vi "Read Settings.vi"(0 "Sequence File Path":path, 5 "Charact type":string="Scalar", 7 "Use Operator Mode":bool=TRUE, 11 "error in":errorcluster) -> (4 "Config File Path":path, 6 "Silent Option Enabled?":bool, 8 "Check Path Expiration?":bool=TRUE, 10 "Use command-line?":bool=TRUE, 13 "Charact By Standard?":bool, 14 "Setting Section Exists?":bool, 15 "error out":errorcluster)   [LabVIEW 2023, in "RFFixtureCharact.Public.lvlib"]
uses:
  RFFixtureCharact.Public.lvlib
  Common/Data Cache/Settings Dictionary/Setting Keys.vi
  Common/RFCalAndFixtureCharact.Common.lvlib
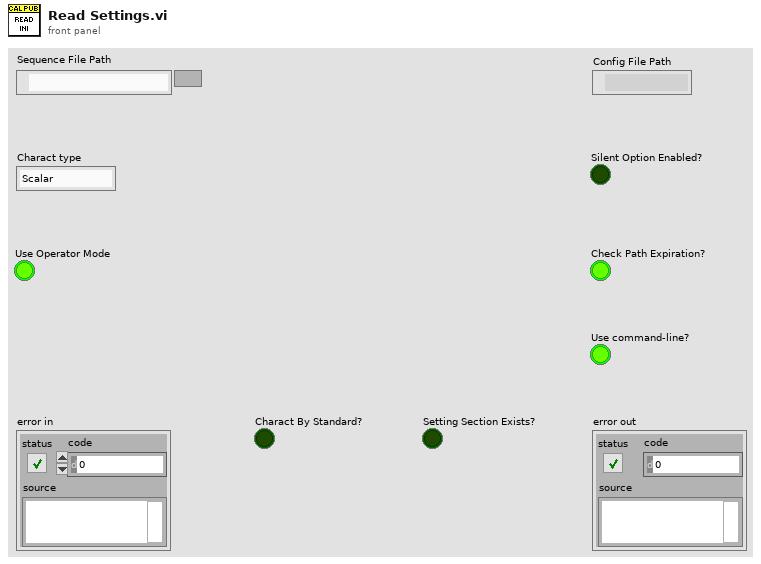
[diagram p1: front panel]
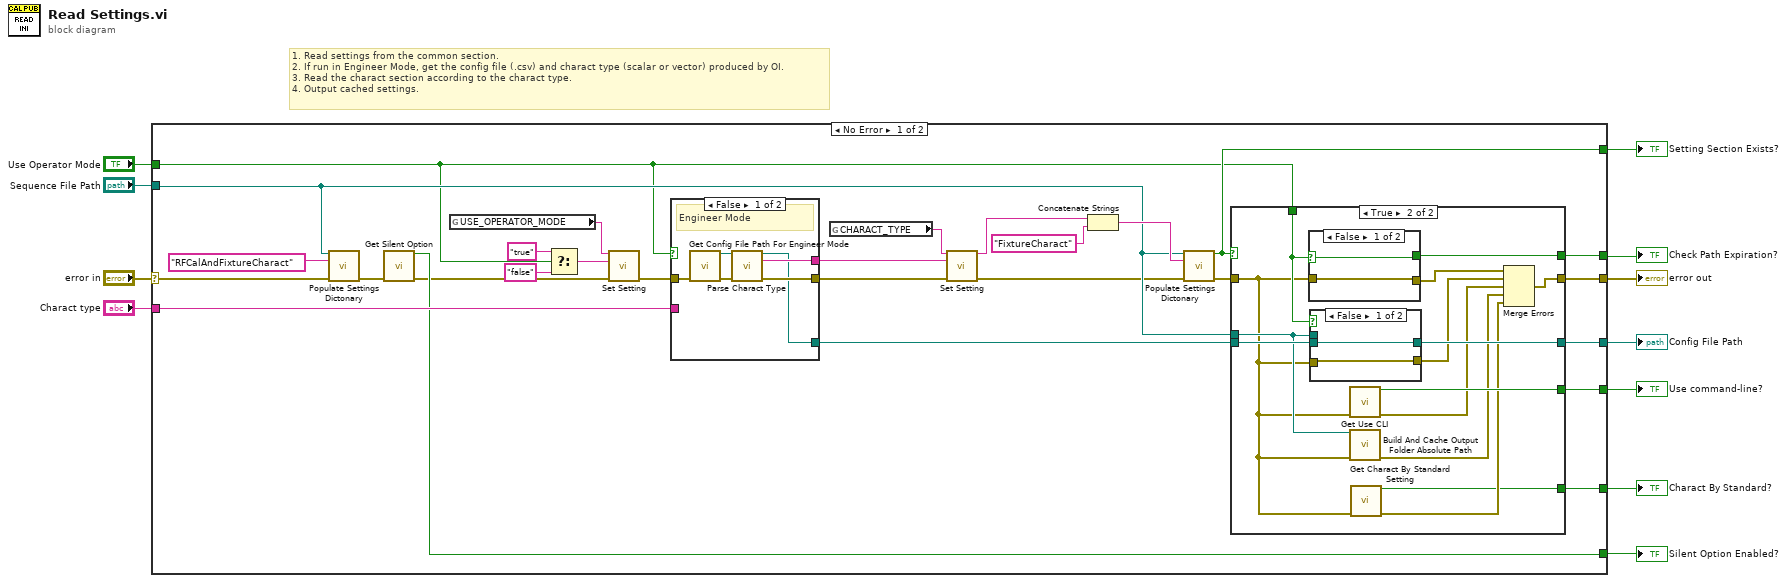
[diagram p0: block diagram]
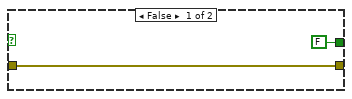
[diagram p2: hidden frame]
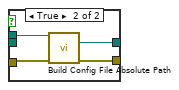
[diagram p3: hidden frame]
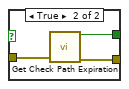
[diagram p4: hidden frame]
diagram:
  # "1. Read settings from the common section.\n2. If run in Engineer Mode, get the config file (.csv) and charact type (scalar or vector) produced by OI.\n3. Read the charact section according to the charact type.\n4. Output cached settings."
  n1 = case shown="No Error" "error in" {
    selector: "error in" -> [w35 w75]
    tunnel: "Charact type" -> [w34 _]
    tunnel: [w19 _] -> w9
    tunnel: [w32 _] -> w8
    tunnel: [w31 _] -> w7
    tunnel: "Sequence File Path" -> [w26 _]
    tunnel: [w30 w75] -> w5
    tunnel: [w33 _] -> w4
    tunnel: [w21 _] -> w3
    tunnel: [w20 _] -> w2
    tunnel: "Use Operator Mode" -> [w15 _]
    frame No Error {
      n2 = call "Populate Settings Dictonary.vi"("sequence file path"=w26, "Section Name"="RFCalAndFixtureCharact", "error in (no error)"=w35) -> ("error out"=w38:errorcluster)  [unwired: 11 in, 1 out]
      n3 = call "Get Silent Option.vi"("error in (no error)"=w38) -> ("Silent Option Enabled?"=w19:bool, "error out"=w18:errorcluster)  [unwired: 13 in]
      n4 = global read "Setting Keys.vi" "USE_OPERATOR_MODE"() -> (w16:string)
      n5 = Select(t="true" ("Section Name"), s=w15, f="false") -> (s? t:f=w12:string)
      n6 = call "Set Setting.vi"("Setting name"=w16, "Setting value"=w12, "error in (no error)"=w18) -> ("error out"=w17:errorcluster)  [unwired: 10 in, 2 out]
      n7 = case shown="False" w15 {
        tunnel: w17 -> [w70 w73]
        tunnel: [w72 w73] -> w36
        tunnel: [w71 w74] -> w24
        tunnel: w34 -> [_ w74]
        tunnel: [w68 _] -> w29
        frame False {
          # "Engineer Mode"
          n8 = call "Get Config File Path For Engineer Mode.vi"("error in (no error)"=w70) -> ("Config File Path"=w67:path, "error out"=w69:errorcluster)  [unwired: 13 in]
          n9 = call "Parse Charact Type.vi"("Config File in"=w67, "error in (no error)"=w69) -> ("Config File out"=w68:path, "Charact type (scalar or vector)"=w71:string, "error out"=w72:errorcluster)  [unwired: 11 in]
        }
        frame True {
          # "Operator Mode"
        }
      }
      n10 = global read "Setting Keys.vi" "CHARACT_TYPE"() -> (w22:string)
      n11 = call "Set Setting.vi"("Setting name"=w22, "Setting value"=w24, "error in (no error)"=w36) -> ("Setting value out"=w23:string, "error out"=w25:errorcluster)  [unwired: 10 in, 1 out]
      n12 = Concatenate Strings(w23, "FixtureCharact" ("string")) -> (w28:string)
      n13 = call "Populate Settings Dictonary.vi"("sequence file path"=w26, "Section Name"=w28, "error in (no error)"=w25) -> ("setting section exists?"=w21:bool, "error out"=w27:errorcluster)  [unwired: 11 in]
      n14 = case shown="True" w21 {
        tunnel: [FALSE ("Check Path Expiration?") w55] -> w33
        tunnel: [_ w54] -> w32
        tunnel: [_ w53] -> w31
        tunnel: [w40 w52] -> w30
        tunnel: w29 -> [_ w48]
        tunnel: w15 -> [_ w47]
        tunnel: w27 -> [w40 w44]
        tunnel: w26 -> [_ w45]
        tunnel: [_ w42] -> w20
        frame False {
        }
        frame True {
          n15 = case shown="False" w47 {
            selector: w47 -> [w63 _]
            tunnel: [w62 w66] -> w51
            tunnel: [w63 w65] -> w55
            tunnel: w44 -> [w62 w64]
            frame False {
            }
            frame True {
              n16 = call "Get Check Path Expiration.vi"("error in (no error)"=w64) -> ("Check Path Expiration?"=w65:bool, "error out"=w66:errorcluster)  [unwired: 13 in]
            }
          }
          n17 = case shown="False" w47 {
            tunnel: [w56 w58] -> w54
            tunnel: w44 -> [w57 w61]
            tunnel: [w57 w60] -> w50
            tunnel: w45 -> [_ w59]
            tunnel: w48 -> [w56 _]
            frame False {
            }
            frame True {
              n18 = call "Build Config File Absolute Path.vi"("Sequence File Path"=w59, "error in (no error)"=w61) -> ("Config File Absolute Path"=w58:path, "error out"=w60:errorcluster)  [unwired: 12 in]
            }
          }
          n19 = call "Get Use CLI.vi"("error in (no error)"=w44) -> ("Use command-lne?"=w53:bool, "error out"=w49:errorcluster)  [unwired: 13 in]
          n20 = call "Build And Cache Output Folder Absolute Path.vi"("Sequence File Path"=w45, "error in (no error)"=w44) -> ("error out"=w46:errorcluster)  [unwired: 13 in]
          n21 = call "Get Charact By Standard Setting.vi"("error in (no error)"=w44) -> ("Charact By Standard?"=w42:bool, "error out"=w43:errorcluster)  [unwired: 13 in]
          n22 = Merge Errors(w51, w50, w49, w46, w43) -> (w52:errorcluster)
        }
      }
    }
    frame Error {
    }
  }
  "error out" <- w5
  "Config File Path" <- w8
  "Use command-line?" <- w7
  "Silent Option Enabled?" <- w9
  "Check Path Expiration?" <- w4
  "Setting Section Exists?" <- w3
  "Charact By Standard?" <- w2
